vi "sendValue.vi"(8 "error in (no error)":errorcluster, 10 "data":variant, 11 "settingsAppliedDomeTcp in":refnum<class "settingsAppliedDomeTcp.lvclass">) -> (0 "error out":errorcluster, 2 "function return":i32, 3 "settingsAppliedDomeTcp out":refnum<class "settingsAppliedDomeTcp.lvclass">)   [LabVIEW 2016, in "SALLV_AtDome_Messaging.lvlib" / "settingsAppliedDomeTcp.lvclass"]
uses:
  settingsAppliedDomeTcp.lvclass
  ts_sallv_AtDome/DataTypes/logevent_settingsAppliedDomeTcp.ctl
  ts_sallv_AtDome/SALLV_AtDome.lvlib
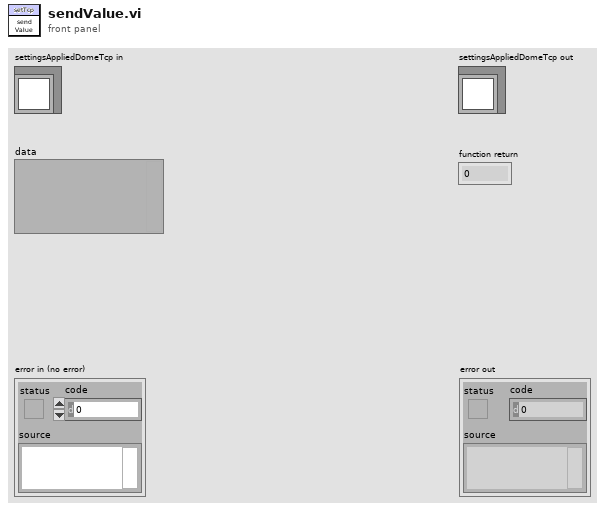
[diagram p1: front panel]
types:
  T1 = typedef "SALLV_AtDome.lvlib/logevent_settingsAppliedDomeTcp.ctl" = cluster{"ip":string, "portRange":i32, "readTimeout":sgl, "writeTimeout":sgl, "connectionTimeout":sgl, "priority":i32}
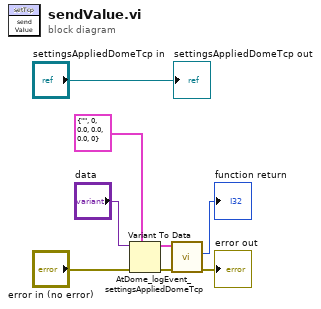
[diagram p0: block diagram]
diagram:
  n1 = Variant To Data(error in="error in (no error)", type=T1 {"ip"="", "portRange"=0, "readTimeout"=0.0, "writeTimeout"=0.0, "connectionTimeout"=0.0, "priority"=0} ("logevent_settingsAppliedDomeTcp_Ctl"), Variant="data") -> (data=w2:T1, error out=w5:errorcluster)
  n2 = call "AtDome_logEvent_settingsAppliedDomeTcp.vi"("error in (no error)"=w5, "logevent_settingsAppliedDomeTcp_Ctl"=w2) -> ("error out"=→"error out":errorcluster, "function return"=→"function return":i32)  [unwired: 7 in, 1 out]
  "settingsAppliedDomeTcp out" <- "settingsAppliedDomeTcp in"
